vi "Communicate - Initialize_Single Device.vi"(8 "error in (no error)":errorcluster, 11 "IP Address":string) -> (0 "error out":errorcluster, 1 "Write Queue Out":refnum<queue>, 2 "Read Queue Out":refnum<queue>, 3 "TCP Network Connection out":refnum<k5>)   [LabVIEW 2020]
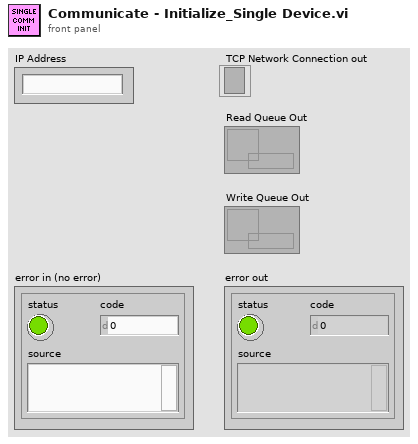
[diagram p1: front panel]
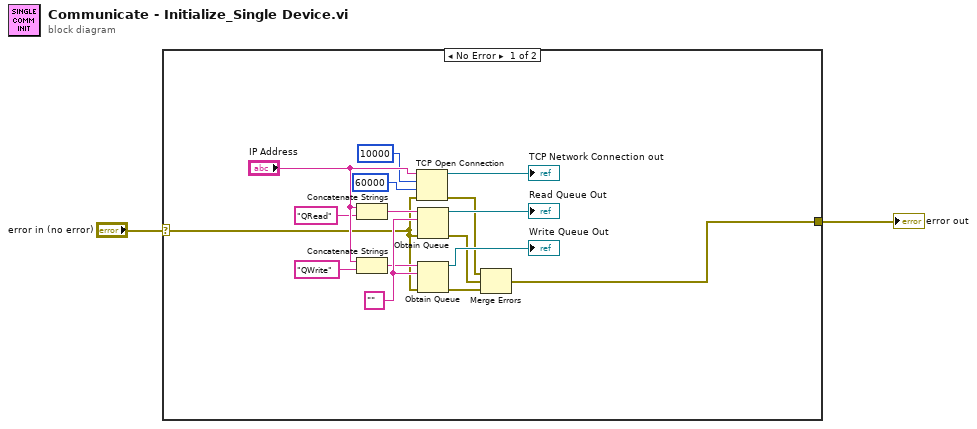
[diagram p0: block diagram]
diagram:
  n1 = case shown="No Error" "error in (no error)" {
    selector: "error in (no error)" -> [w3 w19]
    tunnel: [w16 w19] -> w2
    frame No Error {
      w10 = ""
      n2 = Concatenate Strings("IP Address", "QRead" ("section")) -> (w9:string)
      n3 = Concatenate Strings("IP Address", "QWrite" ("section")) -> (w8:string)
      n4 = TCP Open Connection(address="IP Address", remote port or service name=u16 10000, timeout ms (60000)=60000, error in (no error)=w3) -> (connection ID=→"TCP Network Connection out":refnum<k5>, error out=w11:errorcluster)  [unwired: 1 in]
      n5 = Obtain Queue(name (unnamed)=w9, element data type=w10, error in (no error)=w3) -> (queue out=→"Read Queue Out":refnum<queue>, error out=w12:errorcluster)  [unwired: 2 in, 1 out]
      n6 = Obtain Queue(name (unnamed)=w8, element data type=w10, error in (no error)=w3) -> (queue out=→"Write Queue Out":refnum<queue>, error out=w13:errorcluster)  [unwired: 2 in, 1 out]
      n7 = Merge Errors(w11, w12, w13) -> (w16:errorcluster)
    }
    frame Error {
    }
  }
  "error out" <- w2
